vi "RT_Velocity mode_Oct 25_R2.vi"() -> ()   [LabVIEW 2018]
uses:
  Type Defs/BL Measurement States.ctl
  <vilib>/Platform/TimedLoop/XDataNode/timing_clust.ctl
  <vilib>/Platform/TimedLoop/XDataNode/nitl_modes.ctl
  <vilib>/Platform/TimedLoop/XDataNode/wakeup.ctl
  <vilib>/FPGAPlugInAG/myRIO-1900/niLvFpga_Open_myRIO-1900.vi
  <vilib>/rvi/interface/common/dynamic/niFpgaDynamicAddResources.vi
  <vilib>/Utility/error.llb/Error Cluster From Error Code.vi
  <vilib>/rvi/errors/niLvFpgaAdjustHostInterfaceError.vi
  <vilib>/FPGAPlugInAG/Dynamic/niLvFpga_Close_Dynamic.vi
  <vilib>/Platform/TimedLoop/XDataNode/XDataNode.xnode
  <vilib>/rvi/interface/nirviOpenFPGA/nirviOpenFPGA.xnode
  UNCC Watt balance Oct19/FPGA Bitfiles/UNCCWattbalanceO_FPGATarget_fpganestedFORW&R_sb-Oe1PDHtY.lvbitx
  FPGA files/fpga_nestedFOR_W&R_ADC_W_2DACs_Write_then_CLK.vi
  <vilib>/rvi/interface/nirviReadWriteControl/nirviReadWriteControl.xnode
  <vilib>/rvi/interface/nirviCloseFPGA/nirviCloseFPGA.xnode
  <vilib>/Platform/TimedLoop/XDataNode/XDNodeRunTimeDep.lvlib
  NiFpgaLv.dll
  <vilib>/rvi/interface/Simulation/niFpgaSimulationCallBeginRW.vi
panel:
  out "Numeric Control":i32
  in  "reset BL":bool
  out "Velocity (m/s)":dbl=0.03333406380742028
  out "BL":dbl=14.310883864096947
  out "Cycles 2":dbl=2.5
  out "Time period 2":dbl=0.03704 format="%.4f"
  out "Amplitude (EMF)":dbl=0.47703991586638894 format="%.6f"
  out "Cycles":dbl=2.0
  out "Time period":dbl=0.037 format="%.4f"
  out "Amplitude (CP)":dbl=0.0001964918899367253 format="%.6f"
  in  "no. data points":u16=500
  in  "Measure":bool
  in  "Period (us)":i64=200
  in  "EMF Gain":dbl=1.0
  in  "offset (V)":dbl format="%#_13g"
  in  "frequency (Hz)":dbl=27.0 format="%#_13g"
  in  "amplitude (V)":dbl=0.4 format="%#_13g"
  in  "Stop Button":bool
  out "raw BL":dbl
  out "?":cluster{dbl, dbl}(graph)={161.59573981109904, -162.80879503181404}
  out "XY Graph - Dark":cluster{dbl[], dbl[]}(graph) caption="XY Graph - dark"
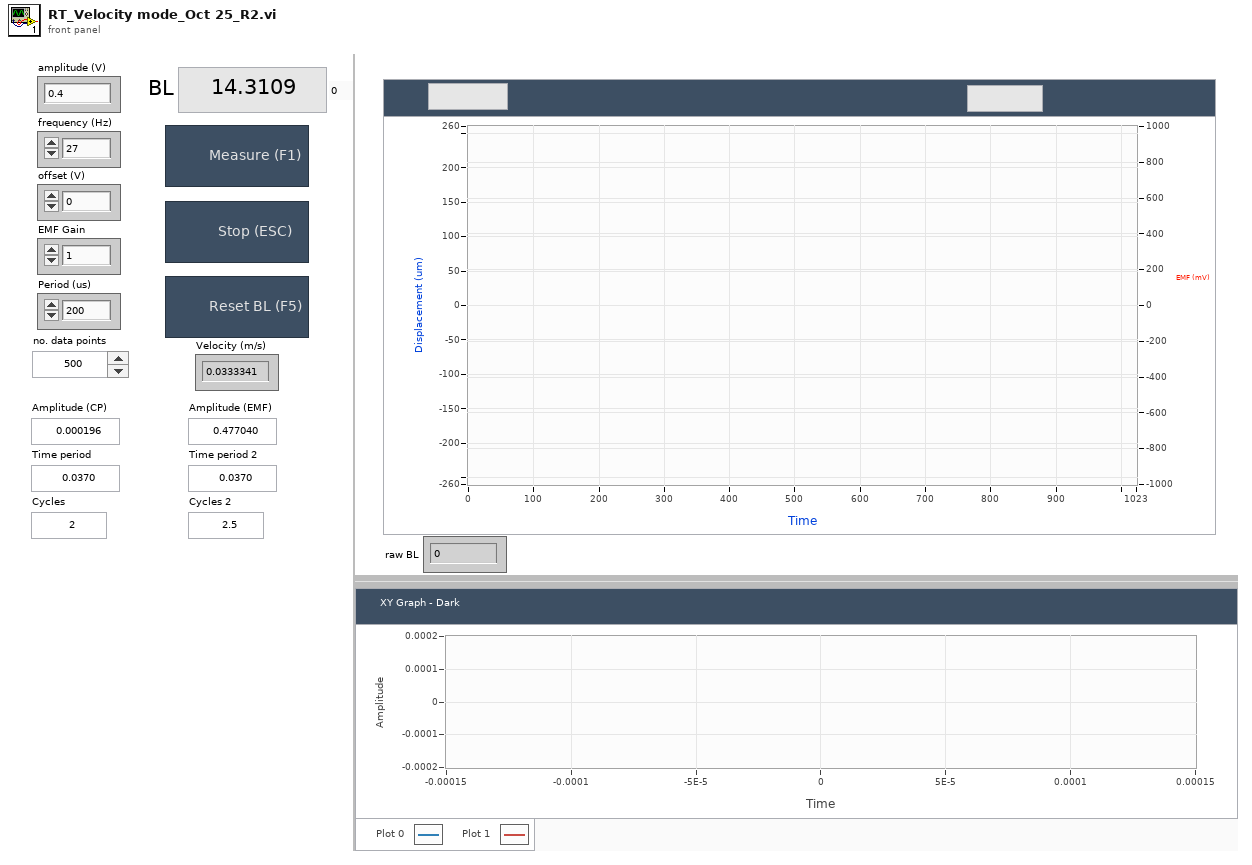
[diagram p1: front panel]
types:
  T1 = typedef "BL Measurement States.ctl" = enum16{"reset BL avg", "idle", "initialize", "collect data", "prepare data", "fit sine", "calculate BL", "exit meas"}
  T2 = typedef "XDNodeRunTimeDep.lvlib/timing_clust.ctl" = cluster{"Expected End [f-1]":u64, "Actual End [f-1]":u64, "Finished Late? [f-1]":bool, "Expected End [i-1]":u64, "Actual End [i-1]":u64, "Finished Late? [i-1]":bool, "Expected Start [i]":u64, "Actual Start [i]":u64, "Expected Start [f]":u64, "Actual Start [f]":u64, "Source Name":string, "Structure Name":string, "Period":i64, "Deadline":i64, "Offset":i64, "Start":i64, "Priority":i32, "Timeout":i32, "Mode":T3, "Wakeup Reason":T4, "Error":errorcluster, "Source Type":string, "Secondary Source Type":string, "Global End Time":u64, "Global Start Time":u64, "Frame Duration":u64, "Iteration Duration":u64, "Assigned CPU":i32, "I/O Scan Engine Mode":u32}
  T3 = typedef "XDNodeRunTimeDep.lvlib/nitl_modes.ctl" = enum32{"No Change", "Process missed periods, maintain original phase", "Discard missed periods, maintain original phase", "Process missed periods, ignore original phase", "Discard missed periods, ignore original phase"}
  T4 = typedef "XDNodeRunTimeDep.lvlib/wakeup.ctl" = enum32{"Normal", "Aborted", "Asynchronous wakeup", "Timing source error", "Timed loop error", "Timeout"}
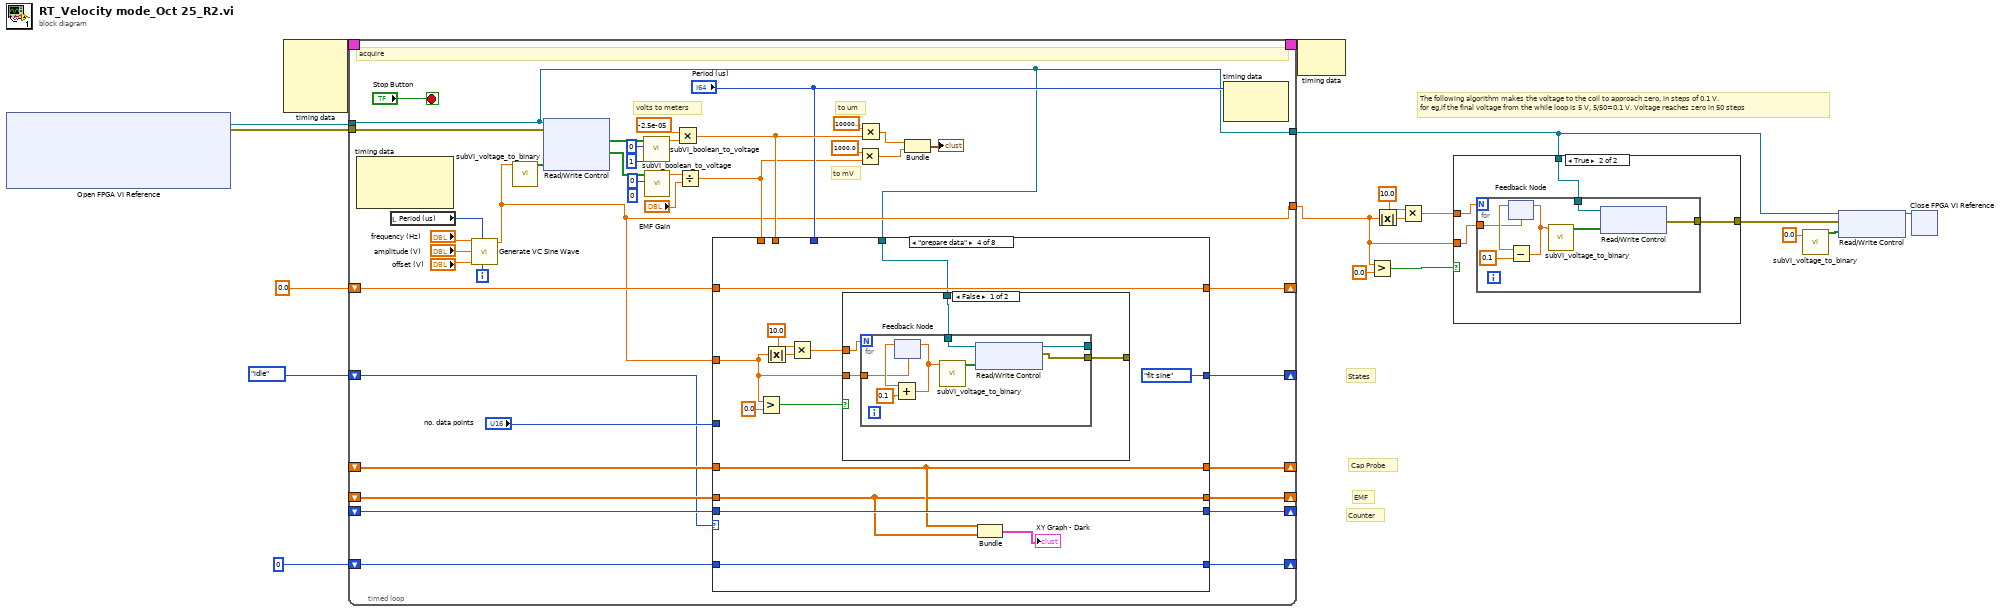
[diagram p0: block diagram]
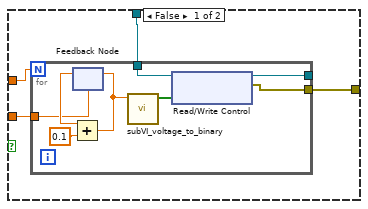
[diagram p2: hidden frame]
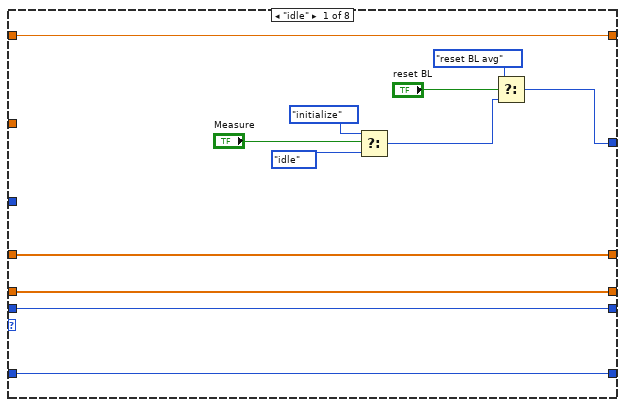
[diagram p3: hidden frame]
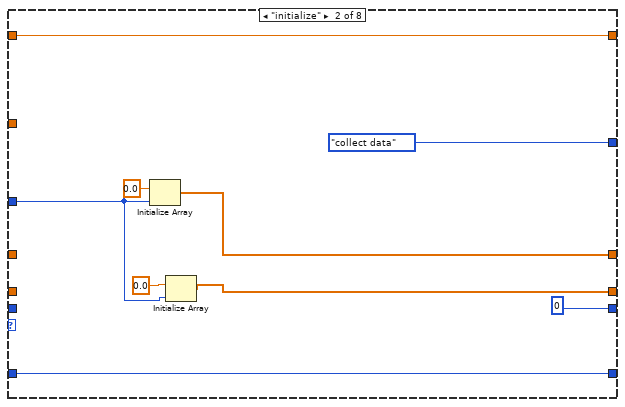
[diagram p4: hidden frame]
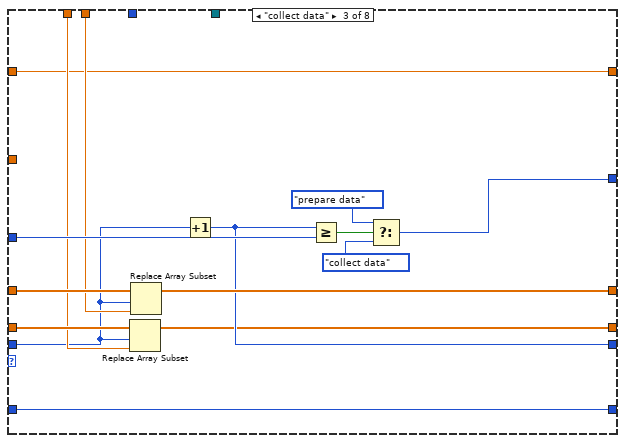
[diagram p5: hidden frame]
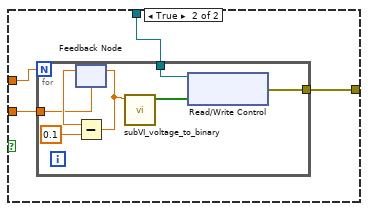
[diagram p6: hidden frame]
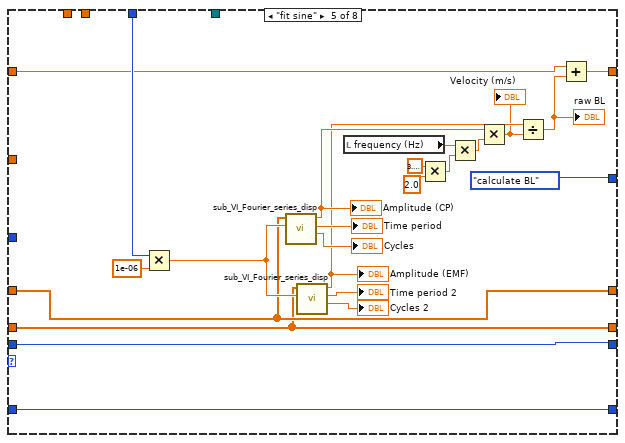
[diagram p7: hidden frame]
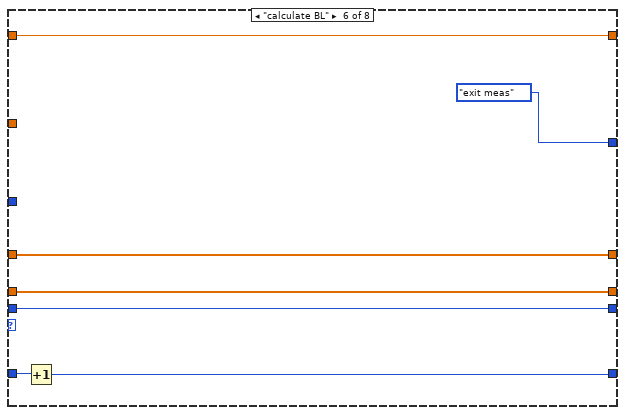
[diagram p8: hidden frame]
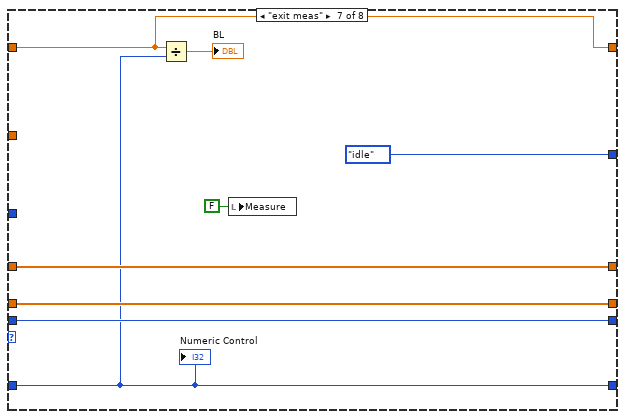
[diagram p9: hidden frame]
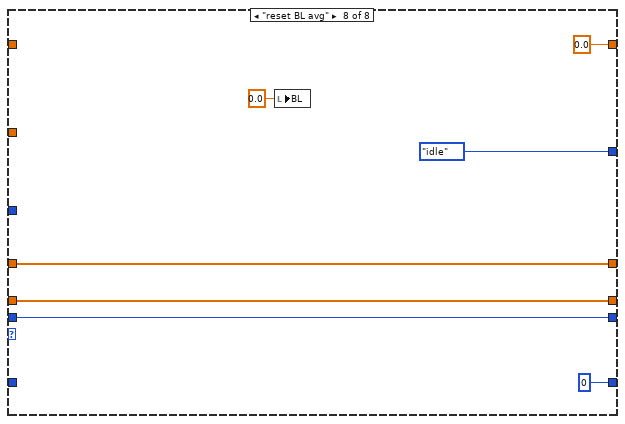
[diagram p10: hidden frame]
diagram:
  # "The following algorithm makes the voltage to the coil to approach zero, in steps of 0.1 V.\nfor eg,if the final voltage from the while loop is 5 V, 5/50=0.1 V. Voltage reaches zero in 50 steps"
  # "States"
  # "Counter"
  # "EMF"
  # "Cap Probe"
  n1 = xnode "Open FPGA VI Reference"() -> ("FPGA VI Reference Out"=w16:refnum<k20>, "error out"=w15:errorcluster)  [unwired: 2 in]
  n2 = node-c288() -> (w18:T2)  [unwired: 4 in]
  n3 = timed-loop {
    timing: w18 -> [_]
    timing-out: [_] -> w17
    tunnel: w16 -> [w19]
    tunnel: w15 -> [w50]
    shift-right: [w44] -> _
    shift-left: BL_Measurement_States."idle" ("BL meas states") -> [w21]
    shift-right: [w43] -> _
    shift-left: _ -> [w42]
    shift-right: [w40] -> _
    shift-left: _ -> [w41]
    shift-right: [w32] -> _
    shift-left: _ -> [w33]
    tunnel: [w20] -> w1
    tunnel: [w19] -> w4
    shift-right: [w25] -> _
    shift-left: 0.0 -> [w24]
    shift-right: [w22] -> _
    shift-left: 0 -> [w23]
    i -> [w58]
    stop <- "Stop Button" stop-if-true
    (unwired) i16 0 ("Gain")
    # "to mV"
    # "to um"
    # "volts to meters"
    # "acquire"
    n4 = node-c288() -> ()  [unwired: 1 in, 3 out]
    n5 = local read "Period (us)"() -> (w54:i64)
    n6 = call "Generate VC Sine Wave.vi"("Counter"=w58, "Period (us)"=w54, "offset (V)"="offset (V)", "amplitude (V)"="amplitude (V)", "frequency (kHz)"="frequency (Hz)") -> ("V"=w20:dbl)  [unwired: 6 in]
    n7 = call "subVI_voltage_to_binary.vi"("voltage"=w20) -> ("binary"=w51:bool[])  [unwired: 10 in]
    n8 = xnode "Read/Write Control"("FPGA VI Reference In"=w19, "error in"=w50, "DAC 1 write"=w51) -> ("ADC  1 R"=w46:bool[], "ADC 2 R"=w45:bool[])  [unwired: 2 out]
    n9 = call "subVI_boolean_to_voltage.vi"("Gain"=i16 1, "UNI"=i16 0, "ADC read"=w46) -> ("V"=w39:dbl)  [unwired: 8 in]
    n10 = call "subVI_boolean_to_voltage.vi"("UNI"=i16 0, "ADC read"=w45) -> ("V"=w38:dbl)  [unwired: 9 in]
    n11 = Multiply(x=-2.5e-05, y=w39) -> (x*y=w37:dbl)
    n12 = Divide(x=w38, y="EMF Gain") -> (x/y=w34:dbl)
    n13 = case shown="\"prepare data\"" w21 {
      tunnel: [w61 BL_Measurement_States."collect data" ("BL meas states") w88 BL_Measurement_States."fit sine" ("BL meas states") BL_Measurement_States."calculate BL" ("BL meas states") BL_Measurement_States."exit meas" ("BL meas states") BL_Measurement_States."idle" ("BL meas states") BL_Measurement_States."idle" ("BL meas states")] -> w44
      tunnel: [w66 w77 w89 w97 w138 w161 w168 w174] -> w43
      tunnel: [w65 w76 w84 w95 w137 w159 w165 w173] -> w32
      tunnel: w42 -> [w66 _ w91 w97 w138 w161 w168 w174]
      tunnel: w41 -> [w67 _ w82 w108 w154 w160 w167 w172]
      tunnel: [w67 0 w86 w108 w154 w160 w167 w172] -> w40
      tunnel: "no. data points" -> [_ w75 w90 _ _ _ _ _]
      tunnel: w37 -> [_ _ w87 _ _ _ _ _]
      tunnel: "Period (us)" -> [_ _ _ _ w151 _ _ _]
      tunnel: w34 -> [_ _ w83 _ _ _ _ _]
      tunnel: w33 -> [w65 _ w85 w95 w137 w159 w165 w173]
      tunnel: [w59 w74 w81 w106 w135 w157 w162 0.0] -> w25
      tunnel: w24 -> [w59 w74 w81 w106 w134 w157 w162 _]
      tunnel: w23 -> [w60 w71 w80 w105 w133 w158 w163 _]
      tunnel: [w60 w71 w80 w105 w133 w156 w163 0] -> w22
      tunnel: w20 -> [_ _ _ w98 _ _ _ _]
      tunnel: w19 -> [_ _ _ w99 _ _ _ _]
      frame "idle" {
        n14 = Select(t=BL_Measurement_States."initialize" ("BL meas states"), s="Measure", f=BL_Measurement_States."idle" ("BL meas states 2")) -> (s? t:f=w62:T1)
        n15 = Select(t=BL_Measurement_States."reset BL avg" ("BL meas states"), s="reset BL", f=w62) -> (s? t:f=w61:T1)
      }
      frame "initialize" {
        n16 = Initialize Array(0.0 ("element"), w75) -> (w77:dbl[])
        n17 = Initialize Array(0.0 ("element"), w75) -> (w76:dbl[])
      }
      frame "collect data" {
        n18 = Replace Array Subset(array=w85, new element=w83, index=w82) -> (w84:dbl[])
        n19 = Replace Array Subset(array=w91, new element=w87, index=w82) -> (w89:dbl[])
        n20 = Increment(x=w82) -> (x+1=w86:i32)
        n21 = Greater Or Equal?(x=w86, y=w90) -> (x >= y?=w92:bool)
        n22 = Select(t=BL_Measurement_States."prepare data" ("BL meas states"), s=w92, f=BL_Measurement_States."collect data" ("BL meas states 2")) -> (s? t:f=w88:T1)
      }
      frame "prepare data" {
        n23 = Greater?(x=w98, y=0.0) -> (0:w100:bool)
        n24 = Absolute Value(x=w98) -> (abs(x)=w104:dbl)
        n25 = Multiply(x=10.0, y=w104) -> (x*y=w101:dbl)
        n26 = case shown="False" w100 {
          tunnel: w101 -> [w112 w124]
          tunnel: w99 -> [w111 w123]
          tunnel: [w110 w122] -> _
          tunnel: w98 -> [w109 w121]
          frame False {
            n27 = for {
              N: w112 -> [_]
              tunnel: [w119] -> _
              tunnel: [w115] -> w110
              tunnel: w111 -> [w114]
              tunnel: w109 -> [w113]
              n28 = feedback #1(w113) -> (w117:dbl)
              n29 = Add(x=w117, y=0.1) -> (x+y=w116:dbl)
              n30 = feedback-in #1(w116) -> ()
              n31 = call "subVI_voltage_to_binary.vi"("voltage"=w116) -> ("binary"=w120:bool[])  [unwired: 10 in]
              n32 = xnode "Read/Write Control"("FPGA VI Reference In"=w114, "DAC 1 write"=w120) -> ("FPGA VI Reference Out"=w119:refnum<k20>, "error out"=w115:errorcluster)  [unwired: 1 in]
            }
          }
          frame True {
            n33 = for {
              N: w124 -> [_]
              tunnel: [w127] -> w122
              tunnel: w123 -> [w126]
              tunnel: w121 -> [w125]
              n34 = feedback #2(w125) -> (w130:dbl)
              n35 = Subtract(x=w130, y=0.1) -> (x-y=w128:dbl)
              n36 = feedback-in #2(w128) -> ()
              n37 = call "subVI_voltage_to_binary.vi"("voltage"=w128) -> ("binary"=w131:bool[])  [unwired: 10 in]
              n38 = xnode "Read/Write Control"("FPGA VI Reference In"=w126, "DAC 2 write"=w131) -> ("error out"=w127:errorcluster)  [unwired: 1 in, 1 out]
            }
          }
        }
        n39 = Bundle(w97, w95) -> (→"XY Graph - Dark":cluster{dbl[], dbl[]})  [unwired: 1 in]
      }
      frame "fit sine" {
        n40 = Multiply(x=w151, y=1e-06) -> (x*y=w140:dbl)
        n41 = call "sub_VI_Fourier_series_disp.vi"("del t"=w140, "x,i"=w138) -> ("number of cycles"=→"Cycles":dbl, "Time period"=→"Time period":dbl, "computed amplitude"=w146:dbl)  [unwired: 6 in, 1 out]
        "Amplitude (CP)" <- w146
        n42 = call "sub_VI_Fourier_series_disp.vi"("del t"=w140, "x,i"=w137) -> ("number of cycles"=→"Cycles 2":dbl, "Time period"=→"Time period 2":dbl, "computed amplitude"=w139:dbl)  [unwired: 6 in, 1 out]
        "Amplitude (EMF)" <- w139
        n43 = local read "frequency (Hz)"() -> (w141:dbl)
        n44 = Multiply(x=3.141592653589793, y=2.0) -> (x*y=w145:dbl)
        n45 = Multiply(x=w141, y=w145) -> (x*y=w142:dbl)
        n46 = Multiply(x=w146, y=w142) -> (x*y=w136:dbl)
        "Velocity (m/s)" <- w136
        n47 = Divide(x=w139, y=w136) -> (x/y=w132:dbl)
        "raw BL" <- w132
        n48 = Add(x=w134, y=w132) -> (x+y=w135:dbl)
      }
      frame "calculate BL" {
        n49 = Increment(x=w158) -> (x+1=w156:i32)
      }
      frame "exit meas" {
        n50 = Divide(x=w162, y=w163) -> (x/y=→"BL":dbl)
        n51 = local write "Measure"(FALSE) -> ()
        "Numeric Control" <- w163
      }
      frame "reset BL avg" {
        n52 = local write "BL"(0.0 ("BL")) -> ()
      }
    }
    n53 = Multiply(x=1000.0, y=w34) -> (x*y=w28:dbl)
    n54 = Multiply(x=1000000.0, y=w37) -> (x*y=w26:dbl)
    n55 = Bundle(w26, w28) -> (→"?":cluster{dbl, dbl})  [unwired: 1 in]
    n56 = node-c288("Period (us)") -> ()  [unwired: 1 in, 1 out]
  }
  n57 = node-c288(w17) -> ()  [unwired: 1 out]
  n58 = Greater?(x=w1, y=0.0) -> (0:w13:bool)
  n59 = Absolute Value(x=w1) -> (abs(x)=w9:dbl)
  n60 = Multiply(x=10.0, y=w9) -> (x*y=w12:dbl)
  n61 = case shown="True" w13 {
    tunnel: w12 -> [w184 w196]
    tunnel: w4 -> [w183 w195]
    tunnel: [w182 w194] -> w5
    tunnel: w1 -> [w181 w193]
    frame False {
      n62 = for {
        N: w184 -> [_]
        tunnel: [w191] -> _
        tunnel: [w187] -> w182
        tunnel: w183 -> [w186]
        tunnel: w181 -> [w185]
        n63 = feedback #3(w185) -> (w189:dbl)
        n64 = Add(x=w189, y=0.1) -> (x+y=w188:dbl)
        n65 = feedback-in #3(w188) -> ()
        n66 = call "subVI_voltage_to_binary.vi"("voltage"=w188) -> ("binary"=w192:bool[])  [unwired: 10 in]
        n67 = xnode "Read/Write Control"("FPGA VI Reference In"=w186, "DAC 1 write"=w192) -> ("FPGA VI Reference Out"=w191:refnum<k20>, "error out"=w187:errorcluster)  [unwired: 1 in]
      }
    }
    frame True {
      n68 = for {
        N: w196 -> [_]
        tunnel: [w199] -> w194
        tunnel: w195 -> [w198]
        tunnel: w193 -> [w197]
        n69 = feedback #4(w197) -> (w202:dbl)
        n70 = Subtract(x=w202, y=0.1) -> (x-y=w200:dbl)
        n71 = feedback-in #4(w200) -> ()
        n72 = call "subVI_voltage_to_binary.vi"("voltage"=w200) -> ("binary"=w203:bool[])  [unwired: 10 in]
        n73 = xnode "Read/Write Control"("FPGA VI Reference In"=w198, "DAC 2 write"=w203) -> ("error out"=w199:errorcluster)  [unwired: 1 in, 1 out]
      }
    }
  }
  n74 = call "subVI_voltage_to_binary.vi"("voltage"=0.0) -> ("binary"=w7:bool[])  [unwired: 10 in]
  n75 = xnode "Read/Write Control"("FPGA VI Reference In"=w4, "error in"=w5, "DAC 1 write"=w7) -> ("FPGA VI Reference Out"=w8:refnum<k20>)  [unwired: 1 out]
  n76 = xnode "Close FPGA VI Reference"("FPGA VI Reference In"=w8) -> ()  [unwired: 1 in, 1 out]
